vi "Get Action 3 Text.vi"(8 "error in":errorcluster, 11 "Plain Parent in":refnum<class "Plain Parent.lvclass">) -> (0 "error out":errorcluster, 2 "Action 3 Text":string, 3 "Plain Parent out":refnum<class "Plain Parent.lvclass">)   [LabVIEW 2021, in "Pop-Up.lvlib" / "Plain Parent.lvclass"]
doc: "data member access VI: read the text of the action 3 button"
uses:
  Plain Parent.lvclass
  Plain Parent.lvclass/Plain Parent.ctl
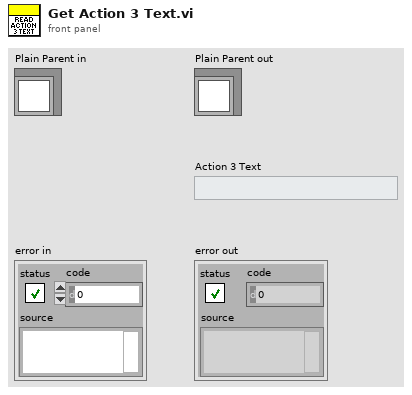
[diagram p1: front panel]
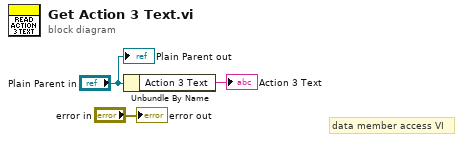
[diagram p0: block diagram]
diagram:
  # "data member access VI"
  n1 = Unbundle By Name("Plain Parent in") -> ("Action 3 Text"=→"Action 3 Text":string)
  "error out" <- "error in"
  "Plain Parent out" <- "Plain Parent in"
